vi "liblinear_predict_values.vi"(8 "error in (no error)":errorcluster, 10 "x":T1[](array[typedef])=[{"index"=0, "value"=0.0}], 11 "liblinear_model":T2={"liblinear_parameter"={"solver_type"=0, "eps"=0.01, "C"=1.0, "weight_label"=[], "weight"=[], "p"=0.1}, "nr_class"=0, "nr_feature"=0, "w"=[], "label"=[], "bias"=0.0} {"liblinear_parameter"."solver_type" items=["L2R_LR"=0, "L2R_L2LOSS_SVC_DUAL"=1, "L2R_L2LOSS_SVC"=2, "L2R_L1LOSS_SVC_DUAL"=3, "MCSVM_CS"=4, "L1R_L2LOSS_SVC"=5, "L1R_LR"=6, "L2R_LR_DUAL"=7, "L2R_L2LOSS_SVR"=11, "L2R_L2LOSS_SVR_DUAL"=12, "L2R_L1LOSS_SVR_DUAL"=13]}) -> (0 "error out":errorcluster, 2 "decision values":dbl[](array[numeric]), 3 "predicted label":dbl)   [LabVIEW 2014]
uses:
  Controls/liblinear_model.ctl
  Controls/liblinear_parameter.ctl
  Controls/liblinear_solver.ctl
  Controls/liblinear_node.ctl
  bin/x64/LVLibSVM.dll
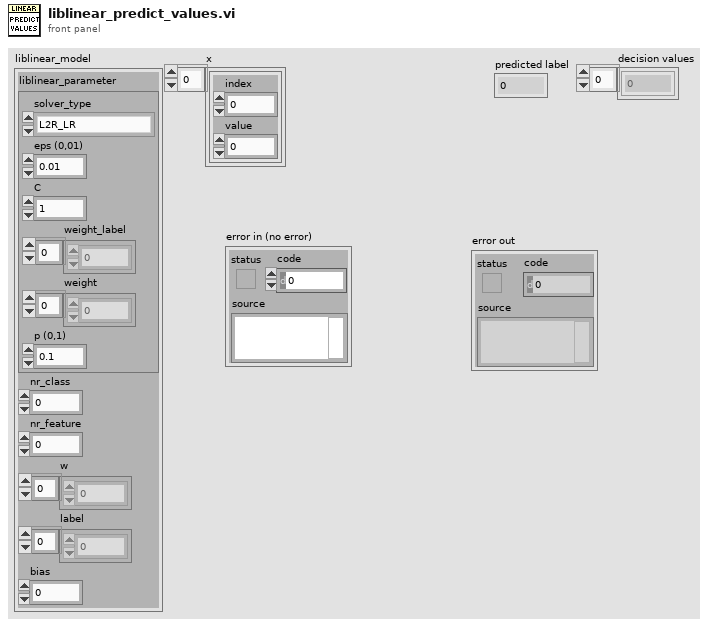
[diagram p1: front panel]
types:
  T1 = typedef "liblinear_node.ctl" = cluster{"index":i32, "value":dbl}
  T2 = typedef "liblinear_model.ctl" = cluster{"liblinear_parameter":T3, "nr_class":i32, "nr_feature":i32, "w":dbl[], "label":i32[], "bias":dbl}
  T3 = typedef "liblinear_parameter.ctl" = cluster{"solver_type":T4, "eps":dbl, "C":dbl, "weight_label":i32[], "weight":dbl[], "p":dbl}
  T4 = typedef "liblinear_solver.ctl" = u32
  T5 = typedef "liblinear_node_padded.ctl" = cluster{"index":i32, "padding":i32, "value":dbl}
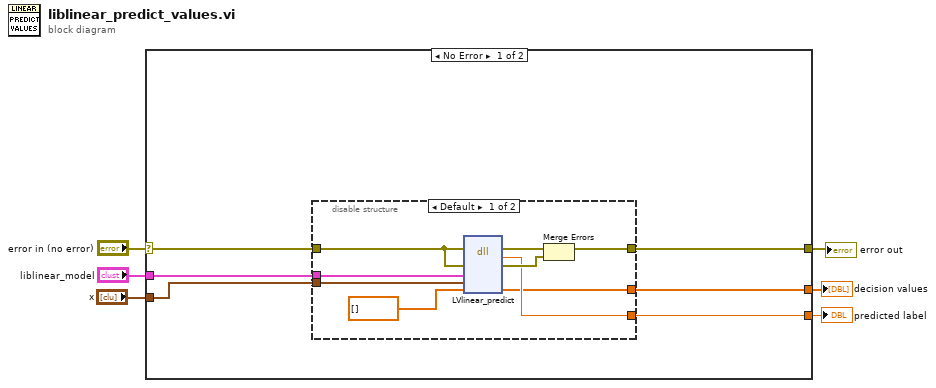
[diagram p0: block diagram]
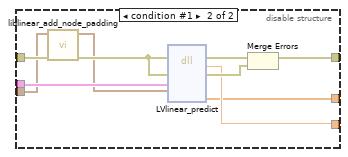
[diagram p2: hidden frame]
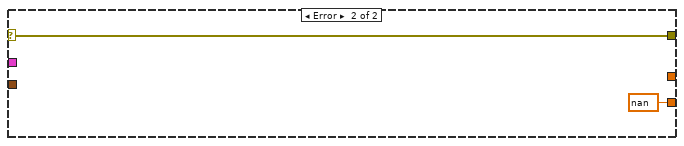
[diagram p3: hidden frame]
diagram:
  n1 = case shown="No Error" "error in (no error)" {
    selector: "error in (no error)" -> [w12 w33]
    tunnel: [w11 w33] -> w6
    tunnel: "liblinear_model" -> [w10 _]
    tunnel: "x" -> [w9 _]
    tunnel: [w8 nan ("predicted label")] -> w2
    tunnel: [w7 _] -> w1
    frame No Error {
      n2 = disable-structure shown="Default" {
        disable-tunnel: w12 -> [w21 w27]
        disable-tunnel: [w19 w30] -> w11
        disable-tunnel: w10 -> [w17 w28]
        disable-tunnel: w9 -> [w16 w25]
        disable-tunnel: [w15 w23] -> w8
        disable-tunnel: [w13 w22] -> w7
        frame condition #0 (active) {
          n3 = dll-call lib="C:/dev/LabVIEW-libsvm/LabVIEW/bin/x64/LVLibSVM.dll" fn="LVlinear_predict"(error in=w21, "lvErr"=w21, "model_in"=w17, "x_in"=w16, "dec_values_out"=dbl[] []) -> (error out=w20:errorcluster, "predicted label"=w15:dbl, "lvErr"=w18:errorcluster, "dec_values_out"=w13:dbl[])  [unwired: 4 in, 1 out]
          n4 = Merge Errors(w20, w18) -> (w19:errorcluster)
        }
        frame condition #1 {
          n5 = call "liblinear_add_node_padding.vi"("error in (no error)"=w27, "Nodes"=w25) -> ("error out"=w26:errorcluster, "Padded nodes"=w24:T5[])  [unwired: 8 in]
          n6 = dll-call lib="C:/dev/LabVIEW-libsvm/LabVIEW/bin/x64/LVLibSVM.dll" fn="LVlinear_predict"(error in=w26, "lvErr"=w26, "model_in"=w28, "x_in"=w24) -> (error out=w31:errorcluster, "predicted label"=w23:dbl, "lvErr"=w29:errorcluster, "dec_values_out"=w22:dbl[])  [unwired: 5 in, 1 out]
          n7 = Merge Errors(w31, w29) -> (w30:errorcluster)
        }
      }
    }
    frame Error {
    }
  }
  "error out" <- w6
  "predicted label" <- w2
  "decision values" <- w1
